vi "Claw Control.vi"(6 "error in (no error)":errorcluster, 7 "Disable Claw Close":bool, 8 "Operation":T9(ring), 9 "MotorControlDevRef":T1={"DeviceStatus"={"status"=FALSE, "code"=0, "source"=""}, "Type"=enum."PWM", "PWM"={"PWM Channel"=enum."Invalid", "DeadBand"={"Name"="", "maxPositivePwm"=0, "minPositivePwm"=0, "centerPwm"=0, "maxNegativePwm"=0, "minNegativePwm"=0, "angularRange"=0}}, "CAN"={"Device Number"=0, "Control Mode"=enum."Percent VBus", "Semaphore"=refnum, "Max Vout"=12.0, "TalonSRX Control Mode"=enum."Percent VBus"}, "Invert"=FALSE, "TransformRef"=refnum, "InvTransformRef"=refnum}) -> (0 "error out":errorcluster, 1 "Holding Open":bool, 2 "Holding":bool, 3 "MotorControlDevRef":T1={"DeviceStatus"={"status"=FALSE, "code"=0, "source"=""}, "Type"=enum."PWM", "PWM"={"PWM Channel"=enum."Invalid", "DeadBand"={"Name"="", "maxPositivePwm"=0, "minPositivePwm"=0, "centerPwm"=0, "maxNegativePwm"=0, "minNegativePwm"=0, "angularRange"=0}}, "CAN"={"Device Number"=0, "Control Mode"=enum."Percent VBus", "Semaphore"=refnum, "Max Vout"=12.0, "TalonSRX Control Mode"=enum."Percent VBus"}, "Invert"=FALSE, "TransformRef"=refnum, "InvTransformRef"=refnum})   [LabVIEW 2015]
uses:
  <vilib>/Rock Robotics/WPI/MotorControl/WPI_MotorControlDeviceRef.ctl
  <vilib>/Rock Robotics/WPI/MotorControl/WPI_MotorControlType.ctl
  <vilib>/Rock Robotics/SystemInterfaces/DIO/FPGA_DIOPWMChannel.ctl
  <vilib>/Rock Robotics/WPI/PWM/WPI_PWMDeadband.ctl
  <vilib>/Rock Robotics/WPI/CAN/Jaguar/SubVIs/WPI_CANJaguar_ControlMode.ctl
  <vilib>/Rock Robotics/WPI/CAN/TalonSRX/WPI_CANTalonSRX_APIControlMode.ctl
  <vilib>/Rock Robotics/WPI/PWM/WPI_PWMTransform_ConPane.ctl
  Robot Global Data.vi
panel:
  in  "Opening time (ms)":u32=400
  in  "Holding Open %VBus":dbl
  in  "Closing time (ms)":u32=420
  in  "Holding %VBus":dbl=0.15
  in  "Opening %VBus":dbl=1.0
  in  "Closing %VBus":dbl=1.0
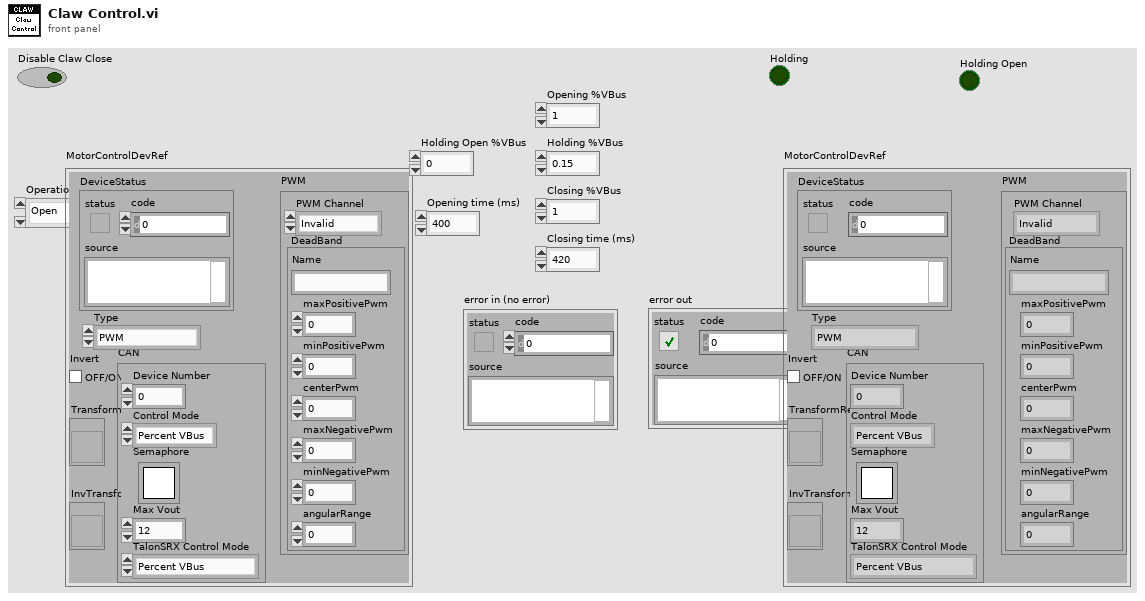
[diagram p1: front panel]
types:
  T1 = typedef "WPI_MotorControlDeviceRef.ctl" = cluster{"DeviceStatus":errorcluster, "Type":T2, "PWM":cluster{"PWM Channel":T3, "DeadBand":T4}, "CAN":cluster{"Device Number":u8, "Control Mode":T5, "Semaphore":T6, "Max Vout":dbl, "TalonSRX Control Mode":T7}, "Invert":bool, "TransformRef":T8, "InvTransformRef":T8}
  T2 = typedef "WPI_MotorControlType.ctl" = enum16{"PWM", "CAN", "CANTalonSRX"}
  T3 = typedef "FPGA_DIOPWMChannel.ctl" = enum8{"PWM 0", "PWM 1", "PWM 2", "PWM 3", "PWM 4", "PWM 5", "PWM 6", "PWM 7", "PWM 8", "PWM 9", "PWM MXP 0", "PWM MXP 1", "PWM MXP 2", "PWM MXP 3", "PWM MXP 4", "PWM MXP 5", "PWM MXP 6", "PWM MXP 7", "PWM MXP 8", "PWM MXP 9", "Invalid"}
  T4 = typedef "WPI_PWMDeadband.ctl" = cluster{"Name":string, "maxPositivePwm":i32, "minPositivePwm":i32, "centerPwm":i32, "maxNegativePwm":i32, "minNegativePwm":i32, "angularRange":u16}
  T5 = typedef "WPI_CANJaguar_ControlMode.ctl" = enum8{"Percent VBus", "Current", "Speed", "Position", "Voltage"}
  T6 = typedef "Semaphore RefNum" = refnum<k1>
  T7 = typedef "WPI_CANTalonSRX_APIControlMode.ctl" = enum8{"Percent VBus", "Speed", "Position", "Slave", "Unchanged / Invalid"}
  T8 = typedef "WPI_PWMTransform_ConPane.ctl" = refnum<vi>
  T9 = enum16{"Open", "Close", "Continue", "Stop", "Toggle"}
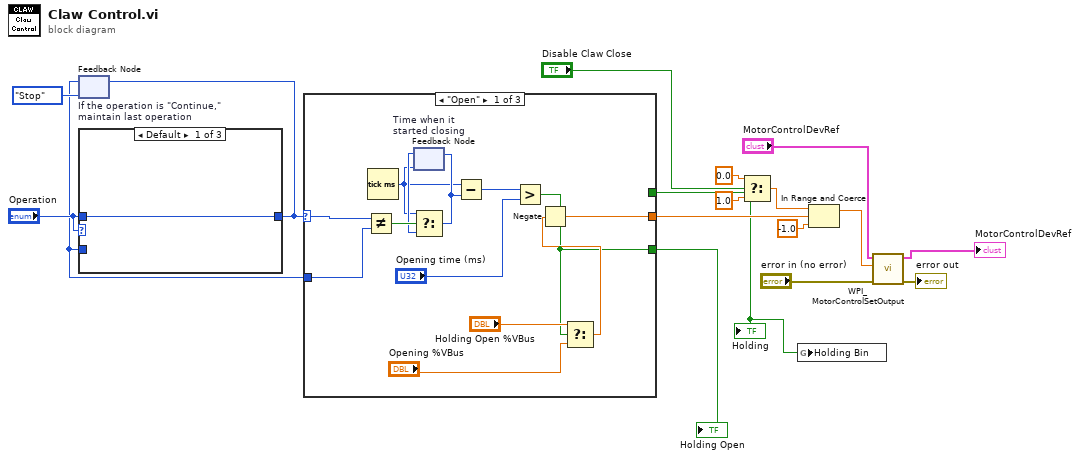
[diagram p0: block diagram]
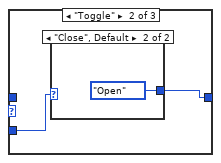
[diagram p2: hidden frame]
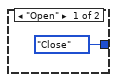
[diagram p3: hidden frame]
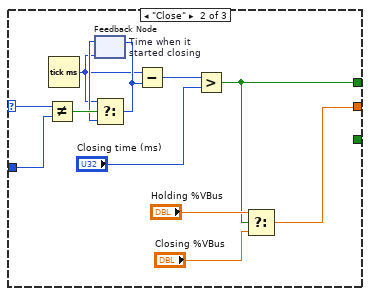
[diagram p5: hidden frame]
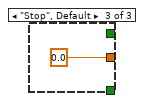
[diagram p6: hidden frame]
diagram:
  n1 = feedback #1 "If the operation is \"Continue,\"\nmaintain last operation"(T9."Stop" ("Operation")) -> (w10:T9)
  n2 = case shown="Default" "Operation" {
    tunnel: [w18 w19 w23] -> w12
    tunnel: w10 -> [_ w20 w23]
    tunnel: "Operation" -> [w18 _ _]
    frame Default {
    }
    frame "Toggle" {
      n3 = case shown="\"Close\", Default" w20 {
        tunnel: [T9."Close" ("Operation") T9."Open" ("Operation")] -> w19
        frame "Open" {
        }
        frame "Close", Default {
        }
      }
    }
    frame "Continue" {
    }
  }
  n4 = feedback-in #1(w12) -> ()
  n5 = case shown="\"Open\"" w12 {
    selector: w12 -> [w26 w46 _]
    tunnel: [w36 w38 0.0 ("Output")] -> w9
    tunnel: w10 -> [w25 w45 _]
    tunnel: [_ w37 _] -> w1
    tunnel: [w24 _ _] -> w2
    frame "Open" {
      n6 = Not Equal?(x=w26, y=w25) -> (x != y?=w34:bool)
      n7 = Tick Count (ms)() -> (millisecond timer value=w31:u32)
      n8 = feedback #2 "Time when it\nstarted closing"(w31) -> (w33:u32)
      n9 = Select(t=w31, s=w34, f=w33) -> (s? t:f=w32:u32)
      n10 = feedback-in #2(w32) -> ()
      n11 = Subtract(x=w31, y=w32) -> (x-y=w30:u32)
      n12 = Greater?(x=w30, y="Opening time (ms)") -> (0:w24:bool)
      n13 = Select(t="Holding Open %VBus", s=w24, f="Opening %VBus") -> (s? t:f=w27:dbl)
      n14 = Negate(x=w27) -> (-x=w36:dbl)
    }
    frame "Close" {
      n15 = Not Equal?(x=w46, y=w45) -> (x != y?=w44:bool)
      n16 = Tick Count (ms)() -> (millisecond timer value=w41:u32)
      n17 = feedback #3 "Time when it\nstarted closing"(w41) -> (w43:u32)
      n18 = Select(t=w41, s=w44, f=w43) -> (s? t:f=w42:u32)
      n19 = feedback-in #3(w42) -> ()
      n20 = Subtract(x=w41, y=w42) -> (x-y=w40:u32)
      n21 = Greater?(x=w40, y="Closing time (ms)") -> (0:w37:bool)
      n22 = Select(t="Holding %VBus", s=w37, f="Closing %VBus") -> (s? t:f=w38:dbl)
    }
    frame "Stop", Default {
    }
  }
  "Holding" <- w1
  "Holding Open" <- w2
  n23 = Select(t=0.0, s="Disable Claw Close", f=1.0) -> (s? t:f=w6:dbl)
  n24 = global write "Robot Global Data.vi" "Holding Bin"(w1) -> ()
  n25 = In Range and Coerce(upper limit=w6, x=w9, lower limit=-1.0) -> (coerced(x)=w8:dbl)  [unwired: 1 out]
  n26 = call <vilib>:"WPI_MotorControlSetOutput.vi"("error in (no error)"="error in (no error)", "Output"=w8, "MotorControlDevRef"="MotorControlDevRef") -> ("error out"=→"error out":errorcluster, "MotorControlDevRef"=→"MotorControlDevRef":T1)  [unwired: 6 in, 1 out]
